vi "ramp.vi"   [LabVIEW 2009]
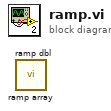
[diagram p0: block diagram]
diagram:
  n1 = call "ramp array.vi"() -> ()  [unwired: 4 in, 2 out]
  n2 = call "ramp dbl.vi"() -> ()  [unwired: 4 in, 2 out]
